vi "INST_PS_SET_VOLTAGE_LEVEL_3.0.0.vi"(4 "Use OPC(T)":bool, 6 "Instrument Select (Output 1)":string(combo), 8 "error in (no error)":errorcluster, 9 "Voltage (0.0)":dbl format="%.2p", 10 "Voltage (0.0)str":string, 11 "VISA session":refnum<visa-resource-name>) -> (0 "error out":errorcluster, 3 "dup VISA session":refnum<visa-resource-name>)   [LabVIEW 2018]
doc: "This VI configures the DC voltage level the power supply attempts to generate.\n\nVer 3.0.0 supports the E36xx Model and The 6634B based on the GPIB address of idtATE [10-12]"
uses:
  Initialize References/Station References Global.vi
panel:
  out "PSn Model":string
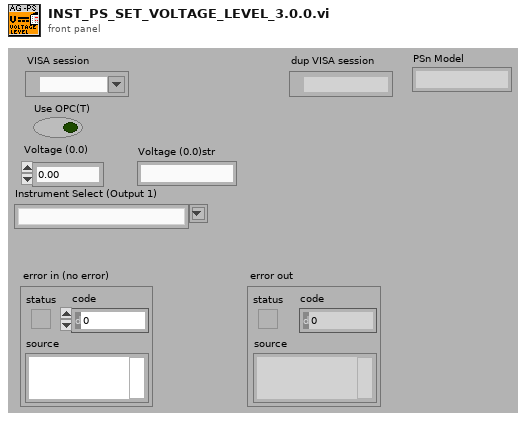
[diagram p1: front panel]
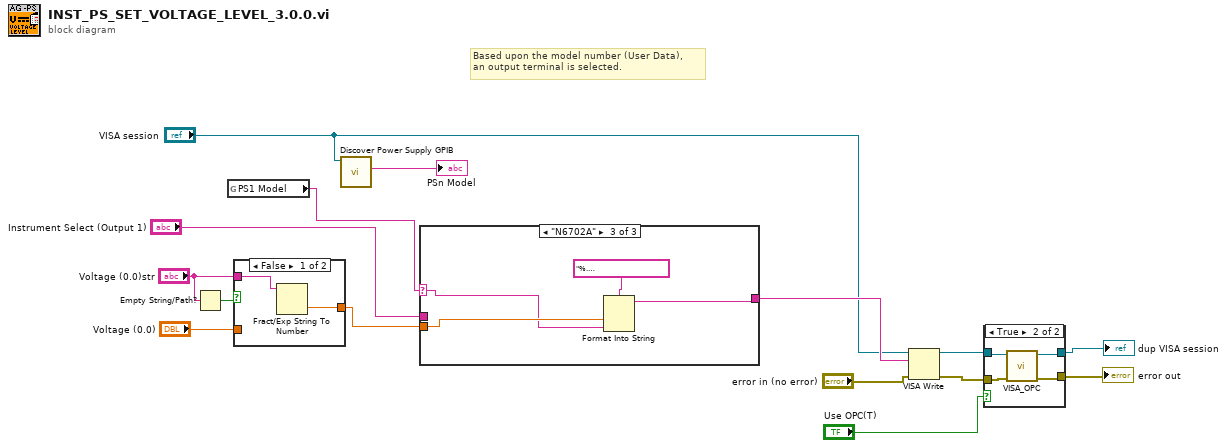
[diagram p0: block diagram]
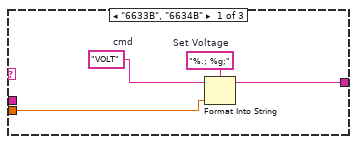
[diagram p2: hidden frame]
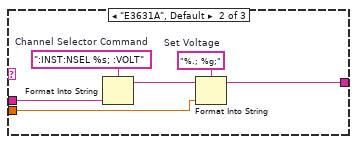
[diagram p3: hidden frame]
diagram:
  # "Based upon the model number (User Data), \nan output terminal is selected."
  n1 = Empty String/Path?(string/path="Voltage (0.0)str") -> (empty?=w7:bool)
  n2 = global read "Station References Global.vi" "PS1 Model"() -> (w1:string)
  n3 = case shown="False" w7 {
    tunnel: "Voltage (0.0)str" -> [w17 _]
    tunnel: [w16 w18] -> w6
    tunnel: "Voltage (0.0)" -> [_ w18]
    frame False {
      n4 = Fract/Exp String To Number(string=w17) -> (number=w16:dbl)  [unwired: 3 in, 1 out]
    }
    frame True {
    }
  }
  n5 = call "Discover Power Supply GPIB.vi"("ADDRESS IN"="VISA session") -> ("PSn Model"=→"PSn Model":string)  [unwired: 10 in]
  n6 = case shown="\"N6702A\"" w1 {
    selector: w1 -> [_ _ w30]
    tunnel: w6 -> [w19 w25 w31]
    tunnel: "Instrument Select (Output 1)" -> [_ w24 _]
    tunnel: [w21 w23 w29] -> w4
    frame "6633B", "6634B" {
      w20 = "VOLT"  # cmd
      w22 = "%.; %g;"  # Set Voltage
      n7 = Format Into String(format string=w22, initial string=w20, w19) -> (resulting string=w21:string)  [unwired: 1 in, 1 out]
    }
    frame "E3631A", Default {
      w26 = ":INST:NSEL %s; :VOLT"  # Channel Selector Command
      w28 = "%.; %g;"  # Set Voltage
      n8 = Format Into String(format string=w26, w24) -> (resulting string=w27:string)  [unwired: 2 in, 1 out]
      n9 = Format Into String(format string=w28, initial string=w27, w25) -> (resulting string=w23:string)  [unwired: 1 in, 1 out]
    }
    frame "N6702A" {
      n10 = Format Into String(format string="%.;SOUR:VOLT:LEV:IMM:AMPL %.;%Le,(@%s)", w31, w30) -> (resulting string=w29:string)  [unwired: 2 in, 1 out]
    }
  }
  n11 = VISA Write(VISA resource name="VISA session", write buffer=w4, error in (no error)="error in (no error)") -> (VISA resource name out=w15:refnum<visa-resource-name>, error out=w14:errorcluster)  [unwired: 1 out]
  n12 = case shown="True" "Use OPC(T)" {
    tunnel: w14 -> [w34 w37]
    tunnel: [w34 w38] -> w11
    tunnel: w15 -> [w33 w36]
    tunnel: [w33 w35] -> w12
    frame False {
    }
    frame True {
      n13 = call "VISA_OPC.vi"("error in"=w37, "Session In"=w36) -> ("error out"=w38:errorcluster, "Session Out"=w35:refnum<visa-resource-name>)  [unwired: 7 in, 1 out]
    }
  }
  "error out" <- w11
  "dup VISA session" <- w12
